vi "_Check if Panther Dashboard is Running.vi"(8 "error in":errorcluster) -> (0 "error out":errorcluster, 3 "Panther Dashboard is Running?":bool)   [LabVIEW 2020, in "Panther Dasboard Scripting Hooks.lvlib"]
uses:
  Panther Dasboard Scripting Hooks.lvlib
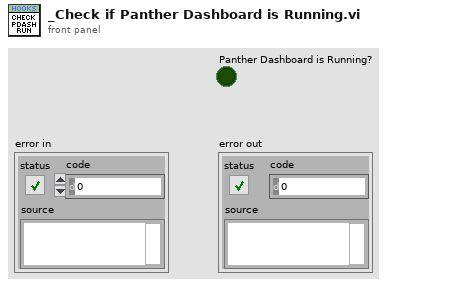
[diagram p1: front panel]
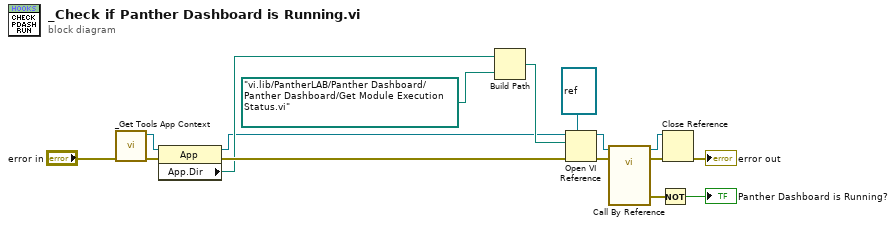
[diagram p0: block diagram]
diagram:
  n1 = call "_Get Tools App Context.vi"("error in"="error in") -> ("error out"=w10:errorcluster, "Application Context"=w1:refnum<vi>)  [unwired: 9 in]
  n2 = property class="App"(reference=w1, error in=w10) -> (reference out=w2:refnum<vi>, error out=w12:errorcluster, "App.Dir"=w4:path)
  n3 = Build Path(base path=w4, name or relative path=path "vi.lib/PantherLAB/Panther Dashboard/Panther Dashboard/Get Module Execution Status.vi") -> (appended path=w6:path)
  n4 = Open VI Reference(type specifier VI Refnum (for type only)=refnum<vi> refnum, application reference (local)=w2, vi path=w6, error in (no error)=w12) -> (vi reference=w7:refnum<vi>, error out=w13:errorcluster)  [unwired: 2 in]
  n5 = call-by-ref "?"(reference=w7, error in=w13) -> (reference out=w8:refnum<vi>, error out=w14:errorcluster, 0:"error out"=w15:errorcluster)  [unwired: 11 in]
  n6 = Not(x=w15) -> (.not. x?=→"Panther Dashboard is Running?":bool)
  n7 = Close Reference(reference=w8, error in (no error)=w14) -> (error out=→"error out":errorcluster)
